vi "autonSample.vi"(0 "Auton Array":dbl[][](array[numeric]), 5 "MeasuredHeading":dbl, 9 "EncoderDistance":dbl) -> (4 "Left Drive":dbl(knob) scale=-1.0..1.0, 6 "Right Drive":dbl(knob) scale=-1.0..1.0, 10 "Turret Rotation":dbl, 14 "Feeder motor":dbl, 15 "Shooter motor output":dbl)   [LabVIEW 2011]
uses:
  Robot Global Data.vi
  <vilib>/addons/control/pid/pid.llb/PID (DBL).vi
  <vilib>/addons/control/pid/NI_PID_pid.lvlib
panel:
  out "Tzero":i64
  out "AccumDist":dbl
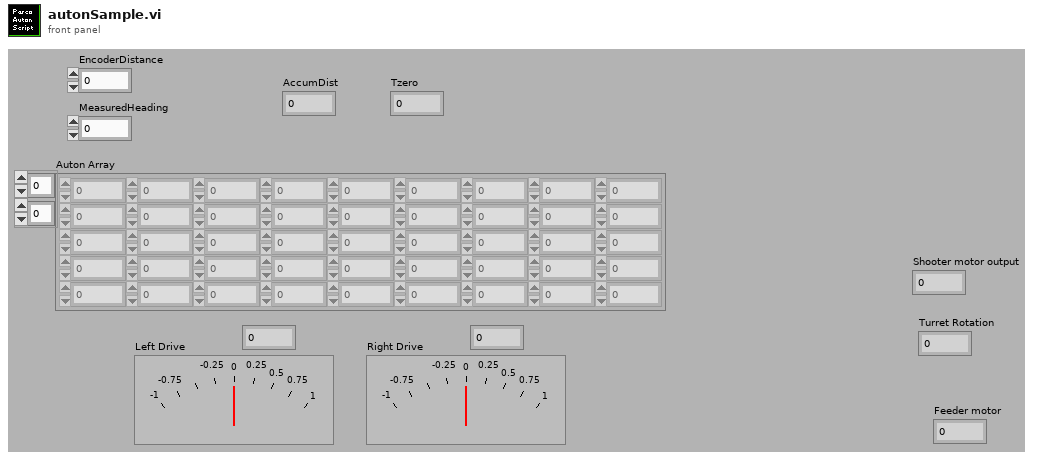
[diagram p1: front panel]
types:
  T1 = cluster{"proportional gain (Kc)":dbl, "integral time (Ti, min)":dbl, "derivative time (Td, min)":dbl}
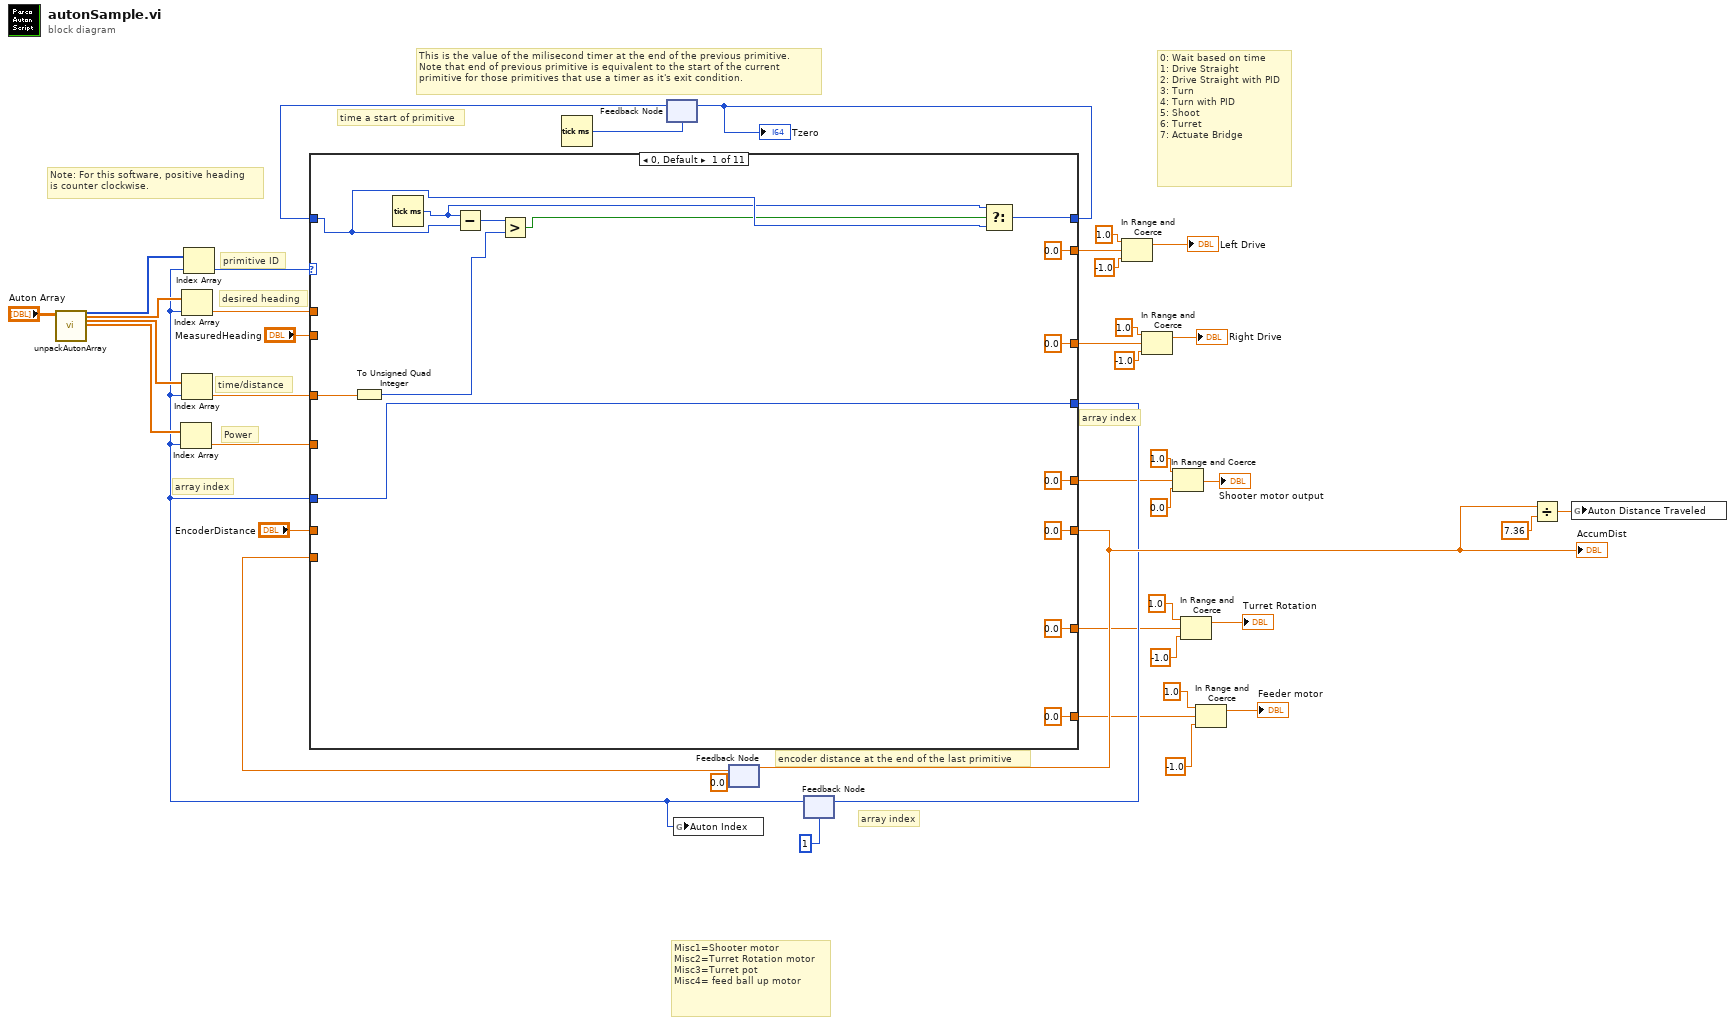
[diagram p0: block diagram]
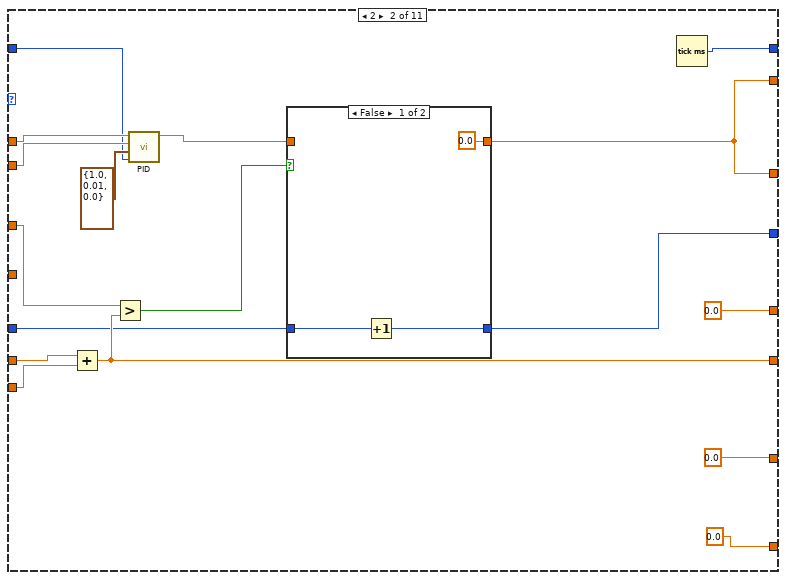
[diagram p2: hidden frame]
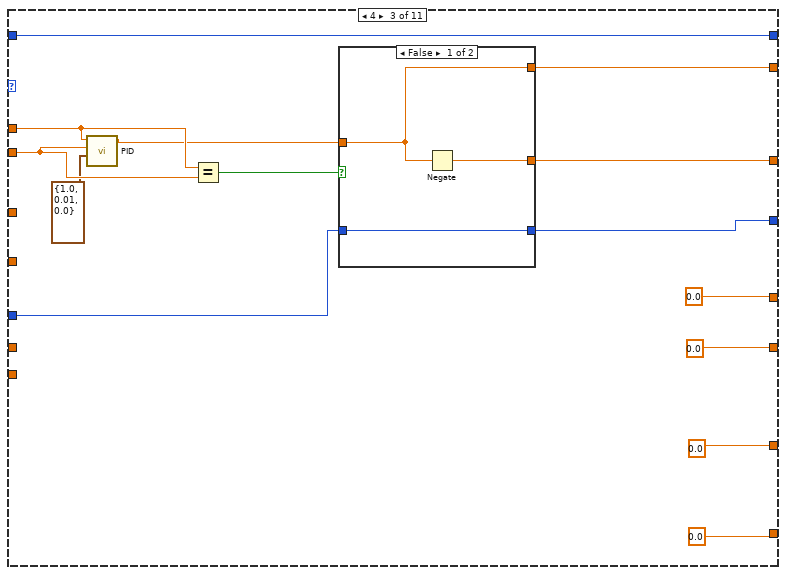
[diagram p4: hidden frame]
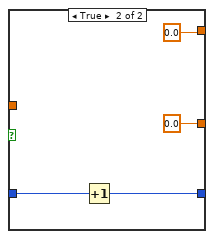
[diagram p5: hidden frame]
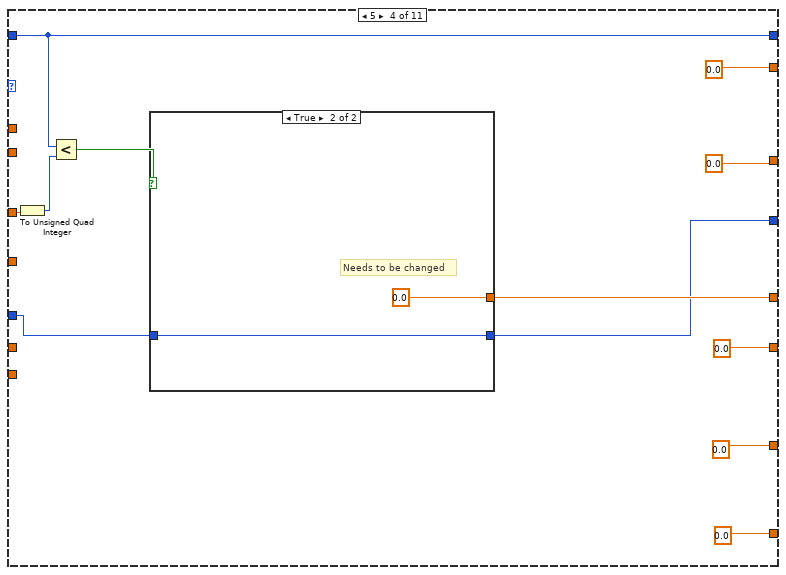
[diagram p6: hidden frame]
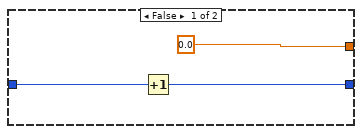
[diagram p7: hidden frame]
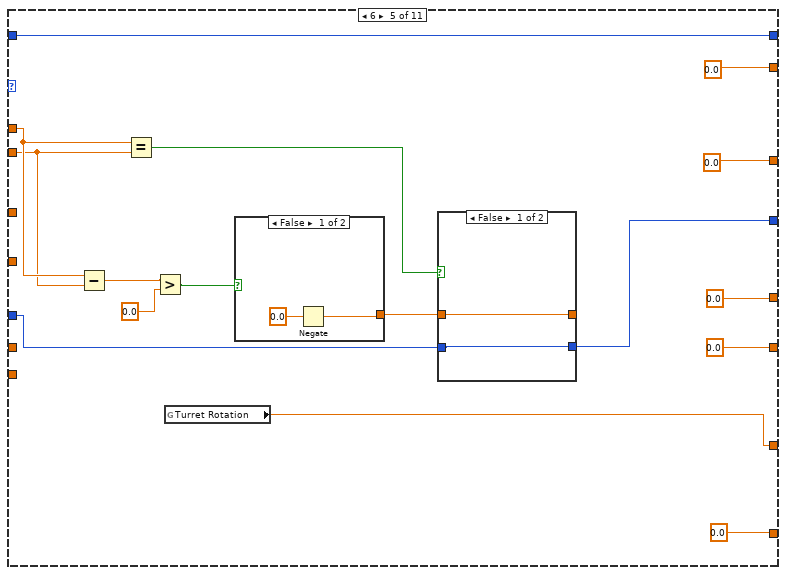
[diagram p8: hidden frame]
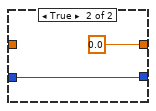
[diagram p9: hidden frame]
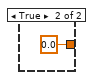
[diagram p10: hidden frame]
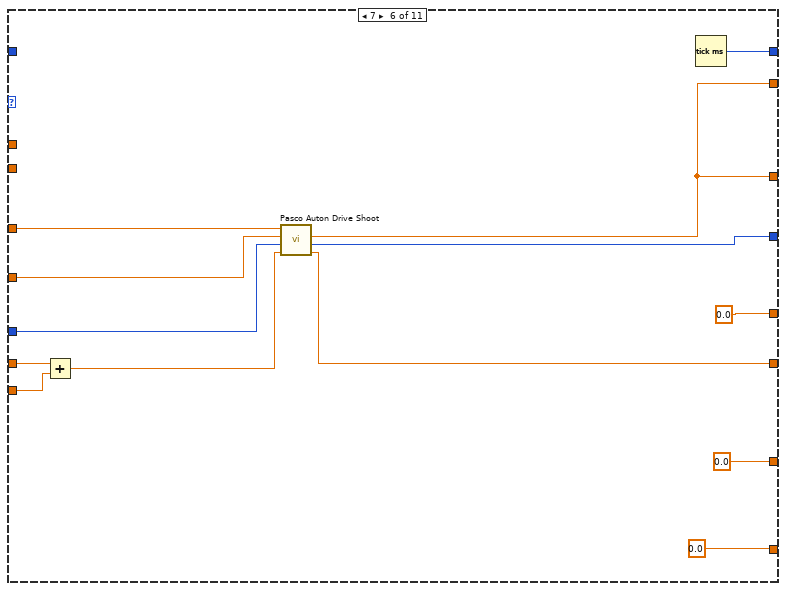
[diagram p11: hidden frame]
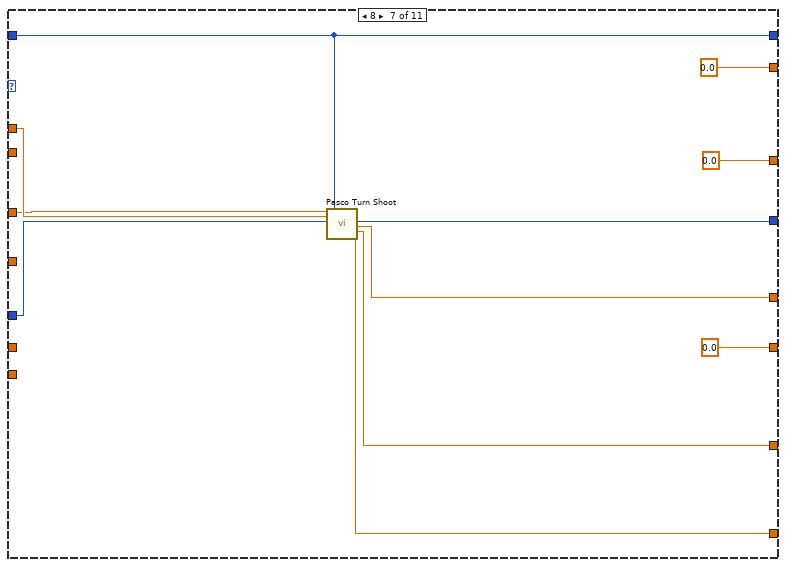
[diagram p12: hidden frame]
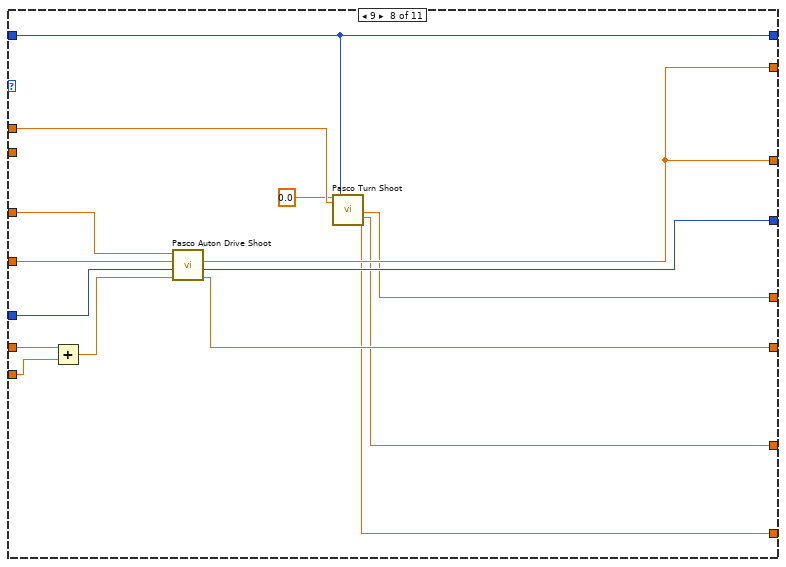
[diagram p13: hidden frame]
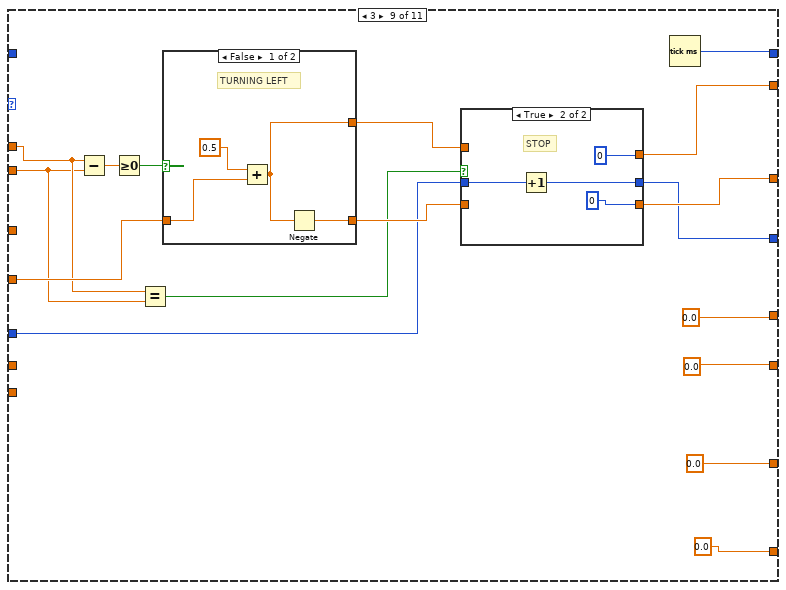
[diagram p14: hidden frame]
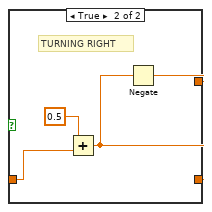
[diagram p16: hidden frame]
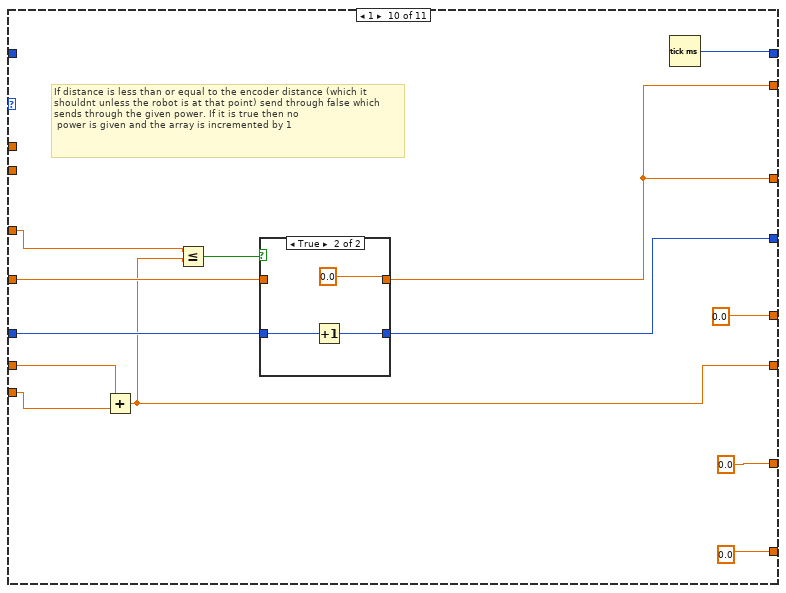
[diagram p17: hidden frame]
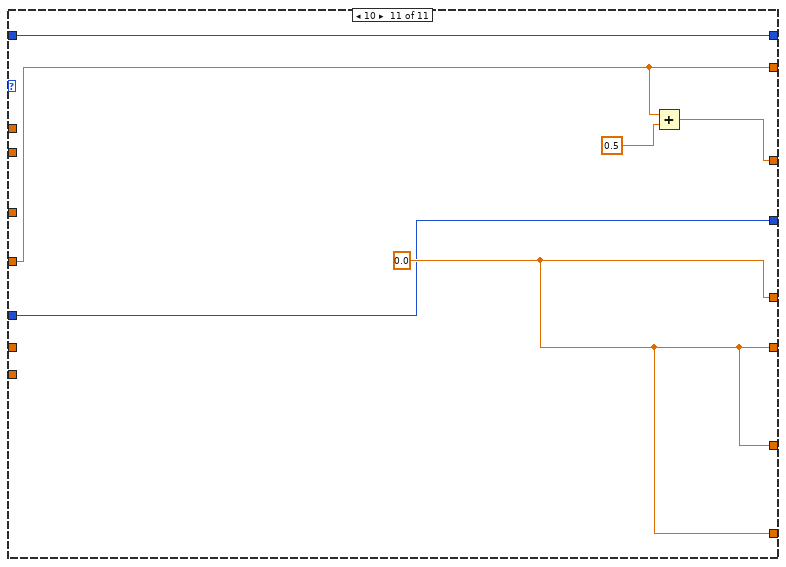
[diagram p19: hidden frame]
diagram:
  # "Misc1=Shooter motor\nMisc2=Turret Rotation motor\nMisc3=Turret pot\nMisc4= feed ball up motor"
  # "0: Wait based on time\n1: Drive Straight\n2: Drive Straight with PID\n3: Turn\n4: Turn with PID\n5: Shoot\n6: Turret\n7: Actuate Bridge"
  # "encoder distance at the end of the last primitive"
  # "Note: For this software, positive heading\nis counter clockwise."
  # "time a start of primitive"
  # "array index"
  # "array index"
  # "This is the value of the milisecond timer at the end of the previous primitive.\nNote that end of previous primitive is equivalent to the start of the current\nprimitive for those primitives that use a timer as it's exit condition."
  # "Power"
  # "array index"
  # "desired heading"
  # "primitive ID"
  # "time/distance"
  n1 = call "unpackAutonArray.vi"("all rows"="Auton Array") -> ("Primitive"=w41:i16[], "Heading"=w23:dbl[], "Distance/Time"=w24:dbl[], "Power"=w21:dbl[])  [unwired: 1 in, 22 out]
  n2 = Tick Count (ms)() -> (millisecond timer value=w35:u32)
  n3 = feedback #1(w35) -> (w39:u32)
  n4 = feedback #2(0.0 ("EncoderDistance")) -> (w20:dbl)
  n5 = feedback #3(1) -> (w2:i32)
  n6 = Index Array(array=w21, index=w2) -> (element=w37:dbl)
  n7 = Index Array(array=w23, index=w2) -> (element=w22:dbl)
  n8 = Index Array(array=w24, index=w2) -> (element=w38:dbl)
  n9 = Index Array(array=w41, index=w2) -> (element=w40:i16)
  n10 = case shown="0, Default" w40 {
    tunnel: [w43 w65 w86 w106 w128 w145 w160 w171 w184 w217 w233] -> w15
    tunnel: w2 -> [w43 w66 w85 w107 w129 w148 w163 w176 w183 w218 w233]
    tunnel: [w56 w73 w92 w101 w127 w141 w161 w166 w190 w216 w232] -> w25
    tunnel: w39 -> [w52 w57 w92 w101 w127 _ w161 w166 _ _ w232]
    tunnel: w38 -> [w54 w69 _ w111 _ w152 w157 w178 _ w221 _]
    tunnel: w22 -> [_ w58 w81 _ w132 _ w162 w170 w192 _ _]
    tunnel: [0.0 ("Numeric") w67 w87 0.0 0.0 w146 0.0 w169 w186 w215 w230] -> w33
    tunnel: [0.0 ("Numeric") w67 w88 0.0 0.0 w146 0.0 w169 w189 w215 w229] -> w26
    tunnel: w37 -> [_ _ _ _ _ w147 _ w177 w194 w219 w230]
    tunnel: "EncoderDistance" -> [_ w72 _ _ _ w151 _ w175 _ w223 _]
    tunnel: "MeasuredHeading" -> [_ w59 w82 _ w118 _ _ _ w191 _ _]
    tunnel: [0.0 ("Encoder total") w70 0.0 0.0 0.0 w144 0.0 w172 0.0 w212 w234] -> w17
    tunnel: w20 -> [_ w71 _ _ _ w150 _ w174 _ w222 _]
    tunnel: [0.0 ("Misc1  OUT") 0.0 0.0 w108 0.0 0.0 ("Misc1  OUT") w159 w168 0.0 0.0 w234] -> w11
    tunnel: [0.0 ("Misc2 OUT") 0.0 0.0 0.0 w117 0.0 ("Misc1  OUT") w158 w167 0.0 0.0 w234] -> w7
    tunnel: [0.0 ("Misc4 OUT") 0.0 0.0 0.0 0.0 0.0 w153 w164 0.0 0.0 w234] -> w3
    frame 0, Default {
      n11 = To Unsigned Quad Integer(1:w54) -> (0:w53:u64)
      n12 = Tick Count (ms)() -> (millisecond timer value=w50:u32)
      n13 = Subtract(x=w50, y=w52) -> (x-y=w55:u32)
      n14 = Greater?(x=w55, y=w53) -> (0:w51:bool)
      n15 = Select(t=w50, s=w51, f=w52) -> (s? t:f=w56:u32)
    }
    frame 2 {
      n16 = Add(x=w72, y=w71) -> (x+y=w70:dbl)
      n17 = Greater?(x=w69, y=w70) -> (0:w68:bool)
      n18 = call-poly <vilib>:"PID.vi"("dt (s)"=w57, "PID gains"=T1 {"proportional gain (Kc)"=1.0, "integral time (Ti, min)"=0.01, "derivative time (Td, min)"=0.0}, "process variable"=w59, "setpoint"=w58) -> ("output"=w61:dbl)  [unwired: 6 in, 1 out]
      n19 = case shown="False" w68 {
        tunnel: [0.0 w78] -> w67
        tunnel: w61 -> [_ w78]
        tunnel: w66 -> [w76 w77]
        tunnel: [w75 w77] -> w65
        frame False {
          n20 = Increment(x=w76) -> (x+1=w75:i32)
        }
        frame True {
        }
      }
      n21 = Tick Count (ms)() -> (millisecond timer value=w73:u32)
    }
    frame 4 {
      n22 = call-poly <vilib>:"PID.vi"("PID gains"=T1 {"proportional gain (Kc)"=1.0, "integral time (Ti, min)"=0.01, "derivative time (Td, min)"=0.0}, "process variable"=w82, "setpoint"=w81) -> ("output"=w80:dbl)  [unwired: 7 in, 1 out]
      n23 = Equal?(x=w81, y=w82) -> (x = y?=w84:bool)
      n24 = case shown="False" w84 {
        tunnel: w80 -> [w94 _]
        tunnel: [w95 0.0] -> w88
        tunnel: [w94 0.0] -> w87
        tunnel: [w93 w98] -> w86
        tunnel: w85 -> [w93 w99]
        frame False {
          n25 = Negate(x=w94) -> (-x=w95:dbl)
        }
        frame True {
          n26 = Increment(x=w99) -> (x+1=w98:i32)
        }
      }
    }
    frame 5 {
      n27 = To Unsigned Quad Integer(1:w111) -> (0:w109:u64)
      n28 = Less?(x=w101, y=w109) -> (x < y?=w110:bool)
      n29 = case shown="True" w110 {
        tunnel: [0.0 0.0] -> w108
        tunnel: w107 -> [w113 w116]
        tunnel: [w112 w116] -> w106
        frame False {
          n30 = Increment(x=w113) -> (x+1=w112:i32)
        }
        frame True {
          # "Needs to be changed"
        }
      }
    }
    frame 6 {
      n31 = Subtract(x=w132, y=w118) -> (x-y=w120:dbl)
      n32 = Equal?(x=w132, y=w118) -> (x = y?=w131:bool)
      n33 = Greater?(x=w120, y=0.0) -> (0:w121:bool)
      n34 = global read "Robot Global Data.vi" "Turret Rotation"() -> (w117:dbl)
      n35 = case shown="False" w121 {
        tunnel: [w138 0.0] -> w130
        frame False {
          n36 = Negate(x=0.0) -> (-x=w138:dbl)
        }
        frame True {
        }
      }
      n37 = case shown="False" w131 {
        tunnel: [w134 0.0] -> _
        tunnel: w130 -> [w134 _]
        tunnel: w129 -> [w133 w136]
        tunnel: [w133 w136] -> w128
        frame False {
        }
        frame True {
        }
      }
    }
    frame 7 {
      n38 = Add(x=w151, y=w150) -> (x+y=w149:dbl)
      n39 = call "Pasco Auton Drive Shoot.vi"("Encoder total"=w149, "Array"=w148, "Power"=w147, "time/distance"=w152) -> ("Encoder total"=w144:dbl, "Array Out"=w145:i32, "Power"=w146:dbl)  [unwired: 5 in]
      n40 = Tick Count (ms)() -> (millisecond timer value=w141:u32)
    }
    frame 8 {
      n41 = call "Pasco Turn Shoot.vi"("time/distance"=w157, "desired heading"=w162, "array index"=w163, "primitive time"=w161) -> ("array index"=w160:i32, "Misc1  OUT"=w159:dbl, "Misc2 OUT"=w158:dbl, "Misc4 OUT"=w153:dbl)  [unwired: 12 in]
    }
    frame 9 {
      n42 = Add(x=w175, y=w174) -> (x+y=w173:dbl)
      n43 = call "Pasco Auton Drive Shoot.vi"("Encoder total"=w173, "Array"=w176, "Power"=w177, "time/distance"=w178) -> ("Encoder total"=w172:dbl, "Array Out"=w171:i32, "Power"=w169:dbl)  [unwired: 5 in]
      n44 = call "Pasco Turn Shoot.vi"("time/distance"=0.0, "desired heading"=w170, "primitive time"=w166) -> ("Misc1  OUT"=w168:dbl, "Misc2 OUT"=w167:dbl, "Misc4 OUT"=w164:dbl)  [unwired: 13 in, 1 out]
    }
    frame 3 {
      n45 = Subtract(x=w192, y=w191) -> (x-y=w195:dbl)
      n46 = Greater Or Equal To 0?(x=w195) -> (x >= 0?=w193:bool)
      n47 = Equal?(x=w192, y=w191) -> (x = y?=w185:bool)
      n48 = case shown="False" w193 {
        tunnel: w194 -> [w205 w207]
        tunnel: [w203 w209] -> w187
        tunnel: [w204 w208] -> w188
        frame False {
          # "TURNING LEFT"
          n49 = Add(x=0.5, y=w205) -> (x+y=w203:dbl)
          n50 = Negate(x=w203) -> (-x=w204:dbl)
        }
        frame True {
          # "TURNING RIGHT"
          n51 = Add(x=0.5, y=w207) -> (x+y=w208:dbl)
          n52 = Negate(x=w208) -> (-x=w209:dbl)
        }
      }
      n53 = case shown="True" w185 {
        tunnel: w183 -> [w198 w202]
        tunnel: [w198 w201] -> w184
        tunnel: [w197 0] -> w189
        tunnel: w188 -> [w197 _]
        tunnel: [w196 0] -> w186
        tunnel: w187 -> [w196 _]
        frame False {
          # "DRIVE"
        }
        frame True {
          # "STOP"
          n54 = Increment(x=w202) -> (x+1=w201:i32)
        }
      }
      n55 = Tick Count (ms)() -> (millisecond timer value=w190:u32)
    }
    frame 1 {
      # "If distance is less than or equal to the encoder distance (which it shouldnt unless the robot is at that point) send through false which sends through the given power. If it is true then no\n power is given and the array is incremented by 1"
      n56 = Add(x=w223, y=w222) -> (x+y=w212:dbl)
      n57 = Less Or Equal?(x=w221, y=w212) -> (x <= y?=w220:bool)
      n58 = case shown="True" w220 {
        tunnel: [w225 0.0] -> w215
        tunnel: w219 -> [w225 _]
        tunnel: w218 -> [w224 w227]
        tunnel: [w224 w226] -> w217
        frame False {
        }
        frame True {
          n59 = Increment(x=w227) -> (x+1=w226:i32)
        }
      }
      n60 = Tick Count (ms)() -> (millisecond timer value=w216:u32)
    }
    frame 10 {
      w234 = 0.0
      n61 = Add(x=w230, y=0.5 ("x+y")) -> (x+y=w229:dbl)
    }
  }
  "AccumDist" <- w17
  "Tzero" <- w25
  n62 = feedback-in #1(w25) -> ()
  n63 = global write "Robot Global Data.vi" "Auton Index"(w2) -> ()
  n64 = feedback-in #2(w17) -> ()
  n65 = feedback-in #3(w15) -> ()
  n66 = In Range and Coerce(upper limit=1.0, x=w33, lower limit=-1.0) -> (coerced(x)=→"Left Drive":dbl)  [unwired: 1 out]
  n67 = In Range and Coerce(upper limit=1.0, x=w26, lower limit=-1.0) -> (coerced(x)=→"Right Drive":dbl)  [unwired: 1 out]
  n68 = In Range and Coerce(upper limit=1.0, x=w11, lower limit=0.0) -> (coerced(x)=→"Shooter motor output":dbl)  [unwired: 1 out]
  n69 = In Range and Coerce(upper limit=1.0, x=w7, lower limit=-1.0) -> (coerced(x)=→"Turret Rotation":dbl)  [unwired: 1 out]
  n70 = In Range and Coerce(upper limit=1.0, x=w3, lower limit=-1.0) -> (coerced(x)=→"Feeder motor":dbl)  [unwired: 1 out]
  n71 = Divide(x=w17, y=7.36) -> (x/y=w1:dbl)
  n72 = global write "Robot Global Data.vi" "Auton Distance Traveled"(w1) -> ()
